vi "Set Subsystem Names.vi"(8 "error in (no error)":errorcluster, 10 "Subsystem Names":string[](array[string]), 11 "Subsystem Controls":refnum<vi>[](array[refnum])) -> (0 "error out":errorcluster, 3 "dup Subsystem Controls":refnum<vi>[](array[refnum]))   [LabVIEW 2024]
doc: "Sets the subsystem names."
uses:
  Controls/Client/Subsystem Overview.ctl
  Controls/Client/Alarm LED.ctl
  Controls/Client/Status LED.ctl
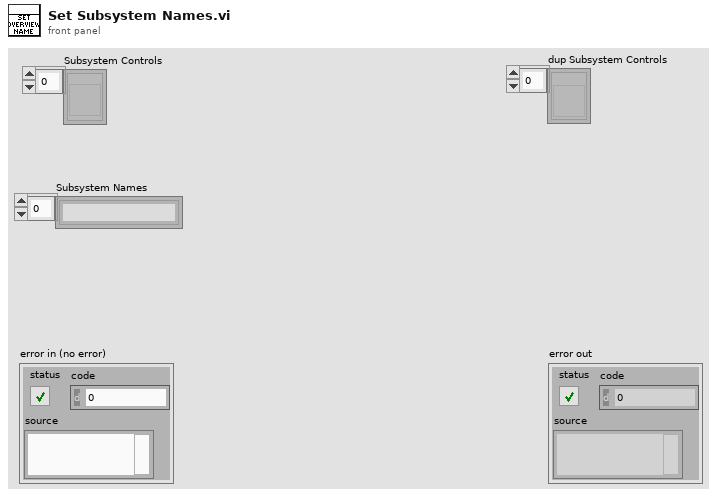
[diagram p1: front panel]
types:
  T1 = typedef "Subsystem Overview.ctl" = cluster{"Subsystem Name":string, "Description":string, "p":dbl, "i":dbl, "d":dbl, "PV":dbl, "SP":dbl, "dt":dbl, "output":dbl, "Alarming?":T2, "In use?":T3}
  T2 = typedef "Alarm LED.ctl" = bool
  T3 = typedef "Status LED.ctl" = bool
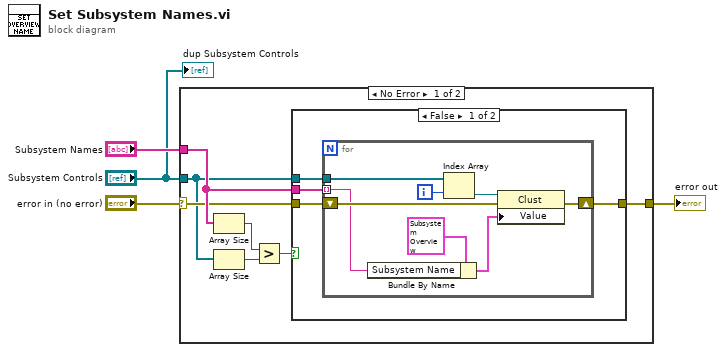
[diagram p0: block diagram]
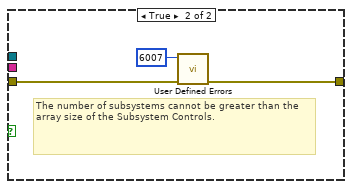
[diagram p2: hidden frame]
diagram:
  n1 = case shown="No Error" "error in (no error)" {
    selector: "error in (no error)" -> [w6 w27]
    tunnel: [w9 w27] -> w3
    tunnel: "Subsystem Names" -> [w7 _]
    tunnel: "Subsystem Controls" -> [w5 _]
    frame No Error {
      n2 = Array Size(array=w7) -> (size(s)=w8:i32)
      n3 = Array Size(array=w5) -> (size(s)=w11:i32)
      n4 = Greater?(x=w8, y=w11) -> (0:w10:bool)
      n5 = case shown="False" w10 {
        tunnel: [w14 w24] -> w9
        tunnel: w7 -> [w15 _]
        tunnel: w6 -> [w13 w25]
        tunnel: w5 -> [w12 _]
        frame False {
          n6 = for {
            shift-right: [w16] -> w14
            shift-left: w13 -> [w18]
            tunnel: w15 -> [w17] mode=indexing
            tunnel: w12 -> [w20]
            i -> [w23]
            n7 = Bundle By Name(cluster=T1 {"Subsystem Name"="", "Description"="", "p"=0.0, "i"=0.0, "d"=0.0, "PV"=0.0, "SP"=0.0, "dt"=0.0, "output"=0.0, "Alarming?"=FALSE, "In use?"=FALSE} ("Value"), "Subsystem Name"=w17) -> (w19:T1)
            n8 = Index Array(array=w20, index=w23) -> (element=w22:refnum<vi>)
            n9 = property class="Clust"(reference=w22, error in=w18, "Value"=w19) -> (error out=w16:errorcluster)  [unwired: 1 out]
          }
        }
        frame True {
          # "The number of subsystems cannot be greater than the array size of the Subsystem Controls."
          n10 = call "User Defined Errors.vi"("error in (no error)"=w25, "Error Code (0)"=6007 ("error code (0)")) -> ("error out"=w24:errorcluster)  [unwired: 9 in]
        }
      }
    }
    frame Error {
    }
  }
  "error out" <- w3
  "dup Subsystem Controls" <- "Subsystem Controls"
